vi "Main_02b.vi"() -> ()   [LabVIEW 2020]
uses:
  ENUM RPS Select.ctl
panel:
  in  "Example":string="A Y\nC Y\nC X\nA Y\nC X\nC Y\nB Z\nA Y\nA Y\nC Z\nA Y\nA Y\nA Y\nC Y\nA Y\nA Y\nA Y\nA X\nB X\nA X\nA Y\nC Y\nC X\nA Y\nA Y\nC Y\nA X\nA Y\nB Z\nA Y\nC X\nA Y\nA Y\nC Z\nC Y\nC X\nA Y\nA Z\nA Y\nA Y\nA Y\nA Y\nC Y\nC Y\nB Z\nB Z\nC Y\nB X\nA Y\nA Y\nA Y\nC Z\nA Y\nC X\nA Z\nC Y\nA Y\nA Y\nA Y\nA Y\nA Y\nC X\nA Y\nC Y\nA Y\nC Y\nA Y\nA X\nC Y\nA X\nA Y\nC Y\nC Y\nA Y\nC X\nA Y\nA Y\nA Y\nC X\nA Y\nA Y\nA Y\nC X\nA Y\nC X\nA Y\nA Y\nC Z\nA Y\nA Y\nA Y\nC X\nA Y\nA X\nC Y\nA X\nB Z\nC Y\nA Y\nA Y\nB Z\nC Y\nA Y\nA Z\nC Z\nC Y\nB Z\nA Y\nA Y\nC Y\nA Y\nC X\nA Y\nA Y\nC X\nC X\nC Y\nA Y\nA Y\nC X\nA Y\nA Y\nA Y\nA Y\nC X\nC Y\nA Y\nA Y\nA Y\nC Z\nA Y\nC Y\nA Y\nC X\nC Z\nA Y\nB X\nA Y\nC X\nA Y\nB X\nA Y\nC Z\nA Y\nA Y\nA Y\nA X\nA Y\nA Y\nA Y\nC Y\nA Y\nA Y\nA Y\nA Y\nC Y\nC X\nA Y\nA Y\nA Y\nA Y\nC Y\nA Y\nA Y\nA Y\nC Y\nB X\nA Y\nA Y\nA Y\nA Y\nA Y\nA X\nC Y\nA Y\nC X\nA X\nB Y\nA Y\nC X\nA Y\nC Y\nC Y\nA Z\nC Z\nC X\nB X\nC Y\nA Y\nC Z\nA Z\nA Y\nC X\nA Y\nA Y\nC X\nA Y\nB X\nC X\nA Z\nC Y\nA Y\nC X\nA Y\nA Y\nA Y\nB Z\nC Z\nA Y\nA X\nC X\nA Y\nA Y\nC Y\nA Y\nA Y\nA X\nA X\nC Y\nC X\nB X\nA Y\nA Y\nA Y\nA Y\nB Y\nA Y\nC Y\nA Y\nA X\nB Z\nA X\nC Z\nC X\nC X\nC Y\nC X\nC X\nA X\nC X\nA Y\nC Y\nA X\nC X\nB Z\nC Z\nA Y\nC X\nB Y\nA Z\nC Y\nC X\nA Y\nA Y\nA Y\nC X\nA Y\nA Y\nA Y\nA X\nB Y\nC Y\nC X\nB Z\nA Y\nA Y\nB Y\nA Y\nA Y\nA Y\nC X\nA Y\nA Y\nA Y\nA Y\nA Y\nA Y\nA Y\nA Y\nA Y\nC Y\nC Y\nC Z\nA Y\nC Y\nA Y\nA Y\nA X\nA X\nA Y\nA Y\nC Y\nA Y\nA X\nA Y\nA Y\nC X\nA Y\nC X\nC X\nC Y\nB Y\nA Y\nC X\nA Y\nA Y\nA X\nA Y\nA Y\nA X\nA Y\nB Z\nC Y\nA Y\nA Y\nA Y\nC Y\nC Z\nA Y\nA Y\nA Y\nA Y\nA Y\nC Y\nC Y\nC Y\nC Y\nC Y\nA X\nC Y\nA Y\nA Y\nA Y\nA Y\nC X\nA Y\nC Z\nA Y\nB Y\nA X\nA Y\nA Y\nA Y\nC Y\nC Y\nA X\nC Y\nA Y\nA Y\nA Y\nB Z\nA X\nA Y\nA Y\nA Z\nC Y\nA Y\nC X\nC Y\nC Y\nC Z\nB Y\nC X\nC X\nA Z\nC Y\nA Y\nA Z\nA X\nA Z\nC Y\nC X\nB Z\nA X\nC Y\nA Y\nC Y\nB Z\nA Y\nA Y\nC X\nC X\nC X\nA Y\nB X\nC X\nC Y\nC X\nA X\nA X\nB X\nA Y\nA Y\nA Y\nC X\nA Y\nC Y\nC X\nA Y\nB Z\nA Y\nA Y\nA Y\nB X\nA Y\nA Y\nA Y\nC Y\nA Y\nC X\nC Y\nC Y\nA Y\nB Z\nC Y\nC X\nC Y\nC X\nC X\nC Y\nA Y\nA Z\nA Y\nA Y\nA Y\nA Y\nC Z\nA Y\nA Y\nC Y\nA Y\nA X\nC Z\nC Y\nC X\nC X\nA Y\nA Z\nA Z\nB Y\nA X\nC X\nC X\nA Y\nA Y\nA Y\nC Z\nC X\nC X\nC X\nA Y\nC Z\nA Z\nC X\nC Y\nA X\nC X\nC X\nA Y\nC Y\nC Y\nB X\nB Z\nA Y\nA Y\nA Y\nB Z\nC Y\nA Y\nB Z\nA X\nC Y\nC Y\nB X\nC X\nB Y\nA Y\nB X\nC Z\nA Y\nA Z\nC Z\nC Z\nA Y\nA X\nA Y\nA X\nC Y\nA Y\nA Y\nA Y\nC X\nC X\nC X\nA Y\nA Y\nA Y\nA Y\nA Y\nC Y\nA Y\nC Y\nA Z\nC X\nC Y\nA Y\nA Y\nB Y\nC Y\nA Y\nC Z\nC Z\nA Y\nB Y\nA Y\nA Y\nA X\nC Y\nA Y\nA Y\nA Y\nC Z\nC Y\nC X\nA Y\nA Y\nB Z\nC Y\nC X\nC Z\nA Y\nC Y\nA Y\nA Y\nC X\nC Y\nC Y\nA Y\nC Y\nC X\nC Y\nA Y\nA Y\nA Y\nA Z\nB Z\nA Y\nA Y\nA X\nC Z\nC X\nA Y\nA Y\nA Y\nC X\nC Y\nB Z\nC X\nA Y\nA Y\nA Y\nC Y\nA Y\nC X\nC Z\nC X\nA Y\nA X\nA Y\nC Z\nC X\nB Y\nA Y\nA X\nA Y\nB Y\nA Y\nA Y\nC Y\nC Z\nC Y\nC Y\nC X\nA Y\nA Y\nA X\nA Y\nA Y\nA Z\nA X\nC Y\nA Y\nC Y\nC Y\nC Z\nC Y\nC Y\nA Z\nA Y\nC Z\nC Y\nC Y\nC Y\nB X\nC Y\nA Y\nC X\nA Y\nB X\nC Z\nC Z\nC Y\nA Y\nC X\nA Y\nA Y\nA Y\nA Y\nC Z\nA Z\nA X\nC Y\nC X\nA Y\nA Y\nC X\nC Y\nC Z\nC X\nC Y\nA X\nA Y\nA Y\nB X\nA Y\nA X\nC X\nA Y\nA Y\nA Y\nB Z\nA Z\nB Z\nC X\nB Z\nA Y\nC X\nA Y\nC X\nA Y\nA Y\nC Y\nA Y\nA Y\nB X\nA Y\nC Y\nA Y\nA Y\nA Y\nC Y\nA Y\nA Y\nA Y\nB Y\nA Y\nC Y\nA Y\nA Y\nA Y\nA Y\nC Y\nA X\nB X\nA Y\nB Z\nC X\nA X\nB X\nC Y\nA Y\nB X\nC Y\nA Y\nB X\nA Y\nC X\nB X\nA Y\nA Y\nA Y\nA Y\nC X\nC X\nA Y\nB X\nC Y\nA Y\nA Y\nA Y\nA Y\nB X\nA Y\nB Z\nC X\nA Y\nB Z\nC X\nC Z\nC Z\nB X\nC Y\nA Y\nA Y\nA Y\nA Y\nA Y\nA Y\nC Y\nA Y\nA Y\nA X\nA X\nC X\nA Y\nC Z\nC Y\nA Y\nC X\nA Z\nA Z\nA Y\nC Z\nA Y\nA Y\nA Y\nC Y\nA X\nC X\nC Z\nA Y\nA Y\nC X\nB X\nA Y\nA Z\nC Y\nA Z\nA Y\nA Y\nA Y\nA Y\nA Y\nB X\nA Y\nC Y\nC X\nA Y\nA Y\nC Z\nC Z\nC Y\nA Y\nB Z\nA Y\nA Y\nA Y\nA Y\nA Y\nC X\nA Z\nA Y\nC Y\nA Z\nC X\nA Y\nC X\nA Y\nA Y\nC Z\nC Y\nA Y\nA Z\nC X\nC X\nA Y\nB Z\nA Y\nB X\nC Y\nC X\nC Z\nA Y\nA X\nC X\nC Z\nC Y\nC X\nA Y\nA Y\nA Y\nA Y\nA Y\nA Y\nC Y\nA Y\nC Y\nA Y\nC Y\nB Y\nA Y\nA Y\nA Y\nA Y\nB Z\nC Y\nA Y\nC Y\nA X\nC Y\nA Y\nB Y\nC Y\nC X\nC X\nA Y\nA Y\nA Y\nC X\nA X\nA Y\nA X\nC Y\nA Y\nA Y\nC Y\nC Y\nA Z\nA Y\nA Y\nB X\nA Z\nB X\nA Y\nC Y\nA X\nC Y\nC Z\nB Z\nA Y\nA Y\nC Y\nA Y\nC Z\nA Y\nA X\nA Y\nC Y\nA Y\nA Y\nA Y\nA Y\nA Y\nA Y\nA Y\nA Y\nC X\nC Y\nA Y\nA Z\nA Y\nC X\nA Y\nC Z\nA Y\nC X\nA X\nA Y\nC Y\nA Y\nC X\nA X\nA Y\nA Y\nA Y\nC Y\nA Y\nC Y\nA Y\nB Y\nC Y\nC Y\nA Y\nA Y\nA Y\nA Y\nC Z\nA Y\nC Z\nA Y\nC Y\nB X\nA X\nC Y\nC Z\nA X\nA Z\nA Y\nA X\nC Z\nC Y\nA Z\nC Y\nA X\nA Y\nA Y\nA X\nC Z\nA X\nA Z\nC Y\nA Y\nC Y\nA Z\nB Z\nA Y\nC X\nC X\nA Y\nA Y\nA X\nA Y\nA Y\nA Y\nC X\nA Y\nB X\nA Y\nC X\nA Y\nC Y\nA Y\nC Y\nC Z\nC Y\nC Z\nA Z\nA Y\nC Y\nC Z\nC Z\nA Y\nA Y\nC Y\nA X\nA Y\nC Y\nA Y\nA Y\nA Y\nA X\nA Y\nB Z\nC Y\nC X\nA Y\nC X\nB X\nC Y\nC Y\nA Y\nC Y\nC Y\nA X\nA Y\nA X\nA Y\nA Z\nC Z\nB X\nA Y\nC X\nA Y\nC Z\nA Y\nC Y\nA Z\nA Y\nA Y\nA Y\nC Y\nC Y\nA Y\nA Y\nC Y\nA Y\nC Y\nC Y\nA X\nA Y\nC X\nC Z\nA Y\nA Y\nA Y\nC X\nC X\nC Y\nC Y\nC Z\nA X\nA Y\nC Y\nC Z\nA Y\nB Y\nA Y\nC Z\nC Z\nA Y\nA Y\nA Y\nB Z\nA Y\nA Z\nA X\nC X\nC X\nC Z\nA Y\nC Z\nA Z\nC Y\nC Z\nC X\nC Y\nC X\nA Y\nC Y\nA Z\nA Y\nA Y\nA Y\nA Y\nC Y\nA X\nC X\nA Y\nA Y\nC Z\nB Z\nA Y\nA Y\nC X\nA Y\nC Y\nC Y\nB Z\nA Y\nC Y\nA Y\nC X\nC X\nA Y\nC Y\nA X\nC X\nA Y\nC Z\nA Y\nC X\nA Y\nC X\nA Y\nC Y\nA Y\nC Z\nA Y\nC Z\nA Y\nA Y\nA Y\nC Y\nA Y\nA X\nA Z\nA Y\nC Y\nC Y\nA Y\nA Y\nB Z\nA X\nA X\nC X\nC X\nC Z\nC Z\nA Y\nA Y\nA Y\nA X\nA X\nA Y\nA Z\nC Y\nC Y\nC X\nA Y\nC X\nB X\nA X\nA Z\nA Y\nB X\nA Y\nB Z\nB Z\nA Y\nB X\nC Y\nA Y\nA Y\nC Y\nC Y\nA Y\nA Y\nA Z\nA Y\nC Z\nB X\nA Y\nC Y\nC Y\nA Y\nB X\nC X\nC Y\nA X\nC X\nA Y\nA X\nA Y\nA Y\nB Z\nA X\nC Y\nA Y\nA Z\nB Y\nA Y\nB X\nA Z\nC Y\nC Z\nC Z\nC Z\nC Y\nA Y\nC Y\nC Y\nB Y\nA Y\nC Z\nB Y\nA Y\nA Y\nA Y\nA X\nB Z\nA Y\nC Z\nA Y\nA X\nC Z\nC X\nA Y\nA Y\nA Y\nB Z\nB Z\nA Y\nC Z\nA Y\nA Y\nA Y\nC Y\nC Z\nC X\nA Y\nB Z\nC Y\nB Z\nC X\nC X\nA Y\nA X\nA X\nB Z\nC Y\nC Y\nC X\nA Y\nC X\nC X\nA Y\nC X\nC Z\nA X\nC Y\nC Y\nC Y\nA Y\nA X\nC Y\nA Y\nA Y\nC Y\nC X\nC Y\nB X\nC X\nA Z\nA X\nA Y\nC Y\nA Y\nA X\nC Y\nA Y\nA X\nC X\nA X\nC X\nC Y\nC Y\nA Y\nC X\nA Y\nA X\nC Y\nA Y\nC Z\nA Z\nA Y\nA Y\nA Y\nA Z\nA Y\nB X\nB Z\nC X\nA Z\nC X\nA Y\nA Z\nA X\nC Y\nC Y\nB Z\nA Z\nA Y\nA Y\nA Y\nB X\nC Y\nA Y\nA X\nA Y\nB Z\nB Z\nA Y\nA Y\nA Y\nC X\nC X\nC X\nC Y\nA Y\nC Y\nC Y\nA Y\nA Y\nA Y\nA Y\nC Y\nA Y\nC X\nA Y\nC X\nC Y\nC Y\nC Z\nB X\nA Y\nC Y\nA Y\nC Y\nA Y\nA Y\nA Y\nA Y\nB Z\nC Z\nC Y\nA X\nC Y\nA Y\nC Y\nC Y\nA Y\nB Z\nC Y\nB X\nB X\nA Y\nA Y\nC Y\nC Y\nB X\nA X\nC Y\nC X\nC Y\nA Y\nA Y\nC X\nA X\nA Z\nA Y\nA Z\nA Y\nB X\nA X\nC X\nA X\nC X\nC Z\nA Y\nC X\nC Y\nC X\nC Y\nA Y\nC Y\nA Y\nA Y\nC Y\nC Z\nC X\nA Y\nA Y\nA X\nC Y\nB Z\nA Y\nC Y\nB Z\nC Y\nA Y\nC Y\nA X\nA X\nA Y\nB X\nA Y\nC X\nC Y\nA Y\nA Y\nA Y\nC X\nC Z\nA Y\nC Y\nA Z\nC Y\nA Y\nC Y\nA Y\nC Z\nC Y\nC X\nA Y\nC X\nA Z\nB Z\nA Y\nA X\nA Y\nA Y\nA X\nA Y\nA Y\nA Y\nA Y\nC Y\nC X\nA Y\nA Y\nA Y\nA Y\nA Y\nC Y\nC Y\nC Y\nA X\nA Z\nA Y\nC X\nA Y\nA Y\nC Y\nB Y\nC Y\nA X\nA Y\nA Y\nA Y\nC X\nA X\nC Y\nC Z\nA Y\nB Z\nA Z\nC Y\nA Y\nA Y\nB Z\nA X\nA Y\nC Y\nA Y\nA X\nB X\nC Z\nB X\nA Y\nA Y\nC Y\nA Y\nA Z\nA Y\nA Y\nA Y\nC X\nA Y\nA Z\nA Z\nA Y\nC X\nA Y\nC Z\nC Y\nB X\nC Y\nA Y\nC Z\nB Z\nA Y\nC Y\nA Z\nA Y\nC X\nC Y\nA X\nA Y\nC Z\nA Y\nA Y\nA Y\nA Y\nB Z\nA Z\nC Z\nA X\nA Y\nA Y\nA Y\nA Y\nA Y\nC Y\nC Y\nA Y\nC X\nA Y\nA Y\nA X\nA X\nA Y\nC Y\nC Z\nA Z\nA Y\nA X\nB X\nB X\nB Z\nC X\nC Y\nA Y\nA Y\nA Y\nC Z\nA Y\nA Y\nA Y\nC Y\nC Y\nB Y\nC Z\nB Z\nC Y\nB Z\nA Y\nA X\nC X\nA X\nC X\nB Y\nA Y\nA Z\nA Y\nA X\nA Y\nA Y\nC X\nA Y\nA Y\nC X\nC X\nA Y\nC X\nC Z\nC X\nB Z\nB Z\nB Z\nC Y\nB Z\nC Y\nC Z\nB Y\nA Y\nC Z\nA Y\nC X\nC X\nB Z\nB Y\nA Y\nA Z\nC Y\nC X\nC Y\nA Z\nC X\nC X\nC X\nA Y\nA Y\nC Y\nA Y\nC Y\nC Y\nA Y\nC Y\nC Z\nA Y\nB Y\nC Y\nC X\nA Y\nA Y\nA X\nA Y\nC Y\nB Z\nA Y\nA Y\nA Y\nA Y\nC X\nB X\nA Y\nA Y\nA Y\nA Y\nB X\nA Y\nA Y\nA X\nC Y\nA Y\nA Y\nC X\nA Y\nA Y\nA Y\nC X\nB Y\nA Z\nC Y\nC X\nA Y\nA Z\nB X\nA Y\nA Y\nA X\nC Y\nC Y\nC Y\nA Y\nC Z\nA Y\nA Y\nC Y\nB Z\nA Y\nA Y\nC X\nA X\nA Y\nA Y\nA Y\nB Z\nC Y\nA Y\nC Y\nC Y\nA Y\nA Y\nC Y\nC Y\nA Y\nC Y\nA Y\nB X\nC Y\nA X\nA Z\nA Y\nA Y\nC Y\nC Y\nA Y\nC Z\nA Z\nA Y\nA Y\nC Y\nC Y\nC X\nC Y\nA Y\nC X\nC Y\nA Y\nC X\nC Y\nC Y\nA Y\nA Y\nA Y\nC X\nC Y\nA Y\nA Y\nC Y\nA Y\nC Y\nA Y\nA Y\nC Y\nC Y\nC Y\nA Z\nA Y\nC Y\nC Y\nA Y\nA X\nC X\nA Y\nC Y\nB X\nC Y\nA Y\nA Y\nC Y\nC Y\nA Y\nA Y\nA Y\nB Z\nA Y\nC Y\nA Y\nA Y\nC X\nC Y\nA Y\nA Y\nC Y\nC Y\nC Y\nC Z\nA Y\nA Y\nC X\nA Y\nC Z\nA X\nC X\nB X\nA Y\nC Y\nA Y\nA Y\nA X\nA Y\nA Z\nB Y\nA X\nA Y\nC Y\nC Y\nC X\nA Y\nC Y\nA Y\nC Y\nA Y\nC X\nC X\nA Y\nC Y\nC Z\nC X\nB X\nA Y\nB X\nA Y\nA Y\nC Y\nA Y\nC Y\nA Y\nA Y\nA Y\nA Y\nA X\nA Z\nA Y\nB X\nA Y\nA Y\nC X\nA Y\nC Z\nA Y\nA Y\nC Y\nC X\nC X\nA Y\nA Y\nB X\nC X\nA Y\nC Y\nA Y\nC Y\nA Y\nB Z\nA Y\nC Y\nA Y\nA Y\nA Y\nC Z\nA Y\nA X\nC X\nA X\nA Y\nA Y\nA Y\nC X\nC Y\nC Y\nC Y\nA Y\nA Y\nA Z\nC X\nA Y\nA Y\nA Y\nC Y\nC Y\nA X\nA Y\nC Y\nB Y\nA Y\nA Z\nC X\nA Y\nA Z\nA X\nA Y\nA Y\nA Y\nC Y\nA Y\nA Y\nA X\nC Y\nA X\nB X\nC X\nC Y\nA Y\nA Y\nA Y\nC Y\nA Y\nA Y\nA Y\nA X\nC X\nA Y\nA Y\nA Y\nC Y\nA Y\nB Y\nC Y\nC Y\nC Y\nC Y\nA Y\nA Y\nC Y\nC Y\nA Y\nC Y\nC Y\nA Y\nC Y\nC X\nC X\nC Y\nA X\nC X\nC X\nA Z\nC Y\nC Z\nA Y\nB Z\nA Y\nA Y\nB X\nC Y\nA Y\nC Z\nA Y\nC Z\nA Y\nA Y\nA X\nC Y\nC X\nC X\nC Y\nC X\nA Y\nA Y\nC X\nA Y\nA Z\nB X\nC X\nC Y\nB X\nB Z\nA Y\nA Y\nA Y\nC Y\nA X\nC Y\nC Y\nC X\nA Y\nC X\nA Y\nA X\nC X\nA Y\nA Y\nA X\nC Y\nB Y\nA Y\nA X\nA Y\nC Y\nA X\nC Y\nA Z\nA Y\nA Y\nC Z\nA Z\nC Y\nA Y\nC Y\nA Y\nA Z\nC Y\nC Y\nB Z\nB Y\nC X\nC X\nB Z\nA Y\nA Y\nA Y\nA Y\nA Y\nA Y\nC X\nA Y\nC Y\nA Y\nB Y\nA Y\nA Y\nB X\nA X\nC X\nC Y\nA Y\nC Y\nA Y\nA Y\nA Y\nA Y\nC X\nB Z\nA Z\nC Y\nB Y\nC X\nA Y\nA X\nA Y\nA Y\nC Y\nC Y\nA Y\nA Y\nC Y\nB Z\nC Y\nA X\nC Y\nA Z\nA Y\nA Y\nA Y\nB X\nA Y\nC Y\nC X\nB Y\nC Y\nA Y\nB Y\nA Y\nA Y\nC X\nC Y\nC Y\nA Y\nA Y\nC X\nC X\nC Y\nA Y\nC X\nC X\nB X\nC Y\nA Y\nC Y\nB Z\nA Y\nB X\nC Y\nC X\nA X\nA Y\nC Y\nA Y\nA Y\nA Y\nC X\nA Y\nC X\nC X\nA Y\nC Y\nA Y\nB Z\nC X\nC Y\nC Y\nB X\nA Y\nC Y\nA X\nA X\nB Z\nC X\nA Y\nC Y\nA Y\nA X\nC Y\nA Y\nA Y\nA X\nA X\nA Z\nC Z\nB Y\nC Y\nC X\nA Y\nA Y\nC Y\nA Y\nC Z\nC X\nC X\nC Z\nC Y\nC X\nC X\nA Y\nC Z\nB X\nC Z\nA Y\nA Y\nC Y\nC X\nC Z\nC X\nC X\nC Y\nC X\nC Y\nA Y\nA X\nA Y\nC X\nA Y\nA Y\nA Y\nA Y\nA Z\nC X\nA X\nB X\nA Y\nA Y\nC Z\nC Y\nA Y\nA Y\nC Y\nC Y\nC Y\nA Y\nA Y\nA Y\nB X\nA Y\nB Z\nA Z\nA X\nA X\nC Y\nA Y\nC Z\nA Y\nA Y\nC Y\nA Y\nA X\nC Y\nC Y\nA X\nA Y\nC Y\nA Y\nC X\nA Y\nC X\nA X\nA Y\nA Y\nA Y\nB X\nC Z\nA Z\nB Y\nA Y\nB Z\nB Z\nA Y\nC Z\nB Z\nA Y\nA Y\nA Y\nC Y\nB X\nA Y\nC X\nA Y\nC Z\nC X\nB Y\nC X\nC X\nB X\nC Y\nB Z\nA X\nA Y\nB Y\nC Z\nA Y\nA Z\nA Y\nC X\nA Y\nA Y\nC Y\nC X\nB Y\nB X\nC Y\nB X\nC Y\nA X\nA Z\nA X\nC X\nB Z\nC Y\nC X\nA Y\nA Y\nA X\nB X\nC X\nA Y\nB Y\nC Z\nA Y\nC Y\nA Y\nA Y\nA Y\nB X\nA Y\nC X\nA Y\nA Y\nA Y\nA X\nC X\nA X\nC Z\nC Y\nA Y\nA Y\nC Y\nA X\nC Z\nA Y\nA Y\nA Y\nB Y\nC Y\nC Y\nC Z\nC Z\nC Z\nA Y\nC Y\nA Y\nA Y\nA Y\nA Y\nA Y\nB Y\nC Y\nC Y\nA X\nC Z\nC Y\nA Y\nA Y\nA Y\nC X\nA Z\nA Y\nA Y\nA X\nA Z\nC X\nB Y\nA Y\nA Y\nC Y\nB X\nA Y\nA Y\nC Y\nC Y\nC Z\nA X\nC Y\nC X\nC X\nC Z\nA X\nB Z\nC X\nC X\nC Y\nC X\nC Z\nC X\nC X\nB Z\nB Z\nA Y\nB Z\nA Y\nA Y\nA Y\nB X\nC X\nA Y\nC Z\nA Z\nA X\nA Y\nB Y\nB X\nB Z\nA Y\nA X\nA X\nA Y\nC X\nB X\nA Y\nC Y\nA Y\nA Y\nC X\nC Y\nC X\nC Z\nB X\nC X\nC Z\nA Z\nA X\nA Y\nA Y\nA Y\nC Z\nA Y\nC Y\nC X\nA Y\nA Y\nC X\nC X\nA Y\nC Y\nC Z\nC Y\nC X\nB Y\nC Y\nC X\nA Y\nB X\nC X\nA Y\nA Y\nC Y\nC Z\nA Y\nA Z\nB Y\nA Y\nB X\nC Y\nC Z\nB X\nB X\nC X\nA Y\nB Z\nA Y\nA Y\nA Y\nA Y\nC X\nA Y\nA Y\nC Z\nC X\nB Y\nC Y\nC Y\nA Y\nC X\nB Z\nA Z\nC Y\nA Y\nB Y\nB X\nB Y\nA Z\nC Y\nC Z\nA Y\nC Z\nC X\nA Y\nA Z\nC Z\nA Y\nA Y\nA Y\nC X\nA Y\nC Y\nB Z\nA Y\nC X\nA X\nA Y\nC Y\nC Z\nC Y\nA Y\nC Z\nA Z\nA Y\nC Y\nA Y\nC X\nA Y\nA Y\nB Z\nA Y\nA Y\nA Y\nC Y\nC Y\nC Y\nC X\nC Y\nC X\nB Z\nA Y\nA Y\nA Z\nA Z\nA Y\nA Z\nA Y\nA Y\nA X\nC Z\nA Y\nA Y\nA Y\nC X\nC Y\nC X\nA Y\nA Y\nA Y\nC Y\nC X\nB Y\nA Y\nC Y\nC Y\nA Z\nC Z\nA Y\nA X\nA Y\nA Y\nB X\nA Y\nC Y\nA X\nC Y\nA Y\nA Y\nA X\nC Y\nA X\nB X\nC Y\nA Y\nA Y\nA Y\nA Y\nC Z\nC Y\nC X\nA X\nA Y\nC X\nC Y\nA X\nA X\nB Y\nB Z\nA Y\nC Z\nA X\nC Y\nA X\nA Y\nC Y\nC X\nC Y\nC X\nA Y\nA X\nA Y\nA X\nC Z\nA X\nA Y\nC Y\nC X\nC Y\nC X\nA Y\nC Y\nC X\nA Y\nA Y\nC Y\nC Y\nA Y\nA Z\nC Y\nA Z\nA Y\nC Y\nA Y\nA Y\nC Y\nA Y\nB X\nC X\nC Y\nC X\nA Y\nB Y\nC Z\nA Y\nC X\nA Y"
  out "Score":u32
  in  "Puzzle":string="A Y\nC Y\nC X\nA Y\nC X\nC Y\nB Z\nA Y\nA Y\nC Z\nA Y\nA Y\nA Y\nC Y\nA Y\nA Y\nA Y\nA X\nB X\nA X\nA Y\nC Y\nC X\nA Y\nA Y\nC Y\nA X\nA Y\nB Z\nA Y\nC X\nA Y\nA Y\nC Z\nC Y\nC X\nA Y\nA Z\nA Y\nA Y\nA Y\nA Y\nC Y\nC Y\nB Z\nB Z\nC Y\nB X\nA Y\nA Y\nA Y\nC Z\nA Y\nC X\nA Z\nC Y\nA Y\nA Y\nA Y\nA Y\nA Y\nC X\nA Y\nC Y\nA Y\nC Y\nA Y\nA X\nC Y\nA X\nA Y\nC Y\nC Y\nA Y\nC X\nA Y\nA Y\nA Y\nC X\nA Y\nA Y\nA Y\nC X\nA Y\nC X\nA Y\nA Y\nC Z\nA Y\nA Y\nA Y\nC X\nA Y\nA X\nC Y\nA X\nB Z\nC Y\nA Y\nA Y\nB Z\nC Y\nA Y\nA Z\nC Z\nC Y\nB Z\nA Y\nA Y\nC Y\nA Y\nC X\nA Y\nA Y\nC X\nC X\nC Y\nA Y\nA Y\nC X\nA Y\nA Y\nA Y\nA Y\nC X\nC Y\nA Y\nA Y\nA Y\nC Z\nA Y\nC Y\nA Y\nC X\nC Z\nA Y\nB X\nA Y\nC X\nA Y\nB X\nA Y\nC Z\nA Y\nA Y\nA Y\nA X\nA Y\nA Y\nA Y\nC Y\nA Y\nA Y\nA Y\nA Y\nC Y\nC X\nA Y\nA Y\nA Y\nA Y\nC Y\nA Y\nA Y\nA Y\nC Y\nB X\nA Y\nA Y\nA Y\nA Y\nA Y\nA X\nC Y\nA Y\nC X\nA X\nB Y\nA Y\nC X\nA Y\nC Y\nC Y\nA Z\nC Z\nC X\nB X\nC Y\nA Y\nC Z\nA Z\nA Y\nC X\nA Y\nA Y\nC X\nA Y\nB X\nC X\nA Z\nC Y\nA Y\nC X\nA Y\nA Y\nA Y\nB Z\nC Z\nA Y\nA X\nC X\nA Y\nA Y\nC Y\nA Y\nA Y\nA X\nA X\nC Y\nC X\nB X\nA Y\nA Y\nA Y\nA Y\nB Y\nA Y\nC Y\nA Y\nA X\nB Z\nA X\nC Z\nC X\nC X\nC Y\nC X\nC X\nA X\nC X\nA Y\nC Y\nA X\nC X\nB Z\nC Z\nA Y\nC X\nB Y\nA Z\nC Y\nC X\nA Y\nA Y\nA Y\nC X\nA Y\nA Y\nA Y\nA X\nB Y\nC Y\nC X\nB Z\nA Y\nA Y\nB Y\nA Y\nA Y\nA Y\nC X\nA Y\nA Y\nA Y\nA Y\nA Y\nA Y\nA Y\nA Y\nA Y\nC Y\nC Y\nC Z\nA Y\nC Y\nA Y\nA Y\nA X\nA X\nA Y\nA Y\nC Y\nA Y\nA X\nA Y\nA Y\nC X\nA Y\nC X\nC X\nC Y\nB Y\nA Y\nC X\nA Y\nA Y\nA X\nA Y\nA Y\nA X\nA Y\nB Z\nC Y\nA Y\nA Y\nA Y\nC Y\nC Z\nA Y\nA Y\nA Y\nA Y\nA Y\nC Y\nC Y\nC Y\nC Y\nC Y\nA X\nC Y\nA Y\nA Y\nA Y\nA Y\nC X\nA Y\nC Z\nA Y\nB Y\nA X\nA Y\nA Y\nA Y\nC Y\nC Y\nA X\nC Y\nA Y\nA Y\nA Y\nB Z\nA X\nA Y\nA Y\nA Z\nC Y\nA Y\nC X\nC Y\nC Y\nC Z\nB Y\nC X\nC X\nA Z\nC Y\nA Y\nA Z\nA X\nA Z\nC Y\nC X\nB Z\nA X\nC Y\nA Y\nC Y\nB Z\nA Y\nA Y\nC X\nC X\nC X\nA Y\nB X\nC X\nC Y\nC X\nA X\nA X\nB X\nA Y\nA Y\nA Y\nC X\nA Y\nC Y\nC X\nA Y\nB Z\nA Y\nA Y\nA Y\nB X\nA Y\nA Y\nA Y\nC Y\nA Y\nC X\nC Y\nC Y\nA Y\nB Z\nC Y\nC X\nC Y\nC X\nC X\nC Y\nA Y\nA Z\nA Y\nA Y\nA Y\nA Y\nC Z\nA Y\nA Y\nC Y\nA Y\nA X\nC Z\nC Y\nC X\nC X\nA Y\nA Z\nA Z\nB Y\nA X\nC X\nC X\nA Y\nA Y\nA Y\nC Z\nC X\nC X\nC X\nA Y\nC Z\nA Z\nC X\nC Y\nA X\nC X\nC X\nA Y\nC Y\nC Y\nB X\nB Z\nA Y\nA Y\nA Y\nB Z\nC Y\nA Y\nB Z\nA X\nC Y\nC Y\nB X\nC X\nB Y\nA Y\nB X\nC Z\nA Y\nA Z\nC Z\nC Z\nA Y\nA X\nA Y\nA X\nC Y\nA Y\nA Y\nA Y\nC X\nC X\nC X\nA Y\nA Y\nA Y\nA Y\nA Y\nC Y\nA Y\nC Y\nA Z\nC X\nC Y\nA Y\nA Y\nB Y\nC Y\nA Y\nC Z\nC Z\nA Y\nB Y\nA Y\nA Y\nA X\nC Y\nA Y\nA Y\nA Y\nC Z\nC Y\nC X\nA Y\nA Y\nB Z\nC Y\nC X\nC Z\nA Y\nC Y\nA Y\nA Y\nC X\nC Y\nC Y\nA Y\nC Y\nC X\nC Y\nA Y\nA Y\nA Y\nA Z\nB Z\nA Y\nA Y\nA X\nC Z\nC X\nA Y\nA Y\nA Y\nC X\nC Y\nB Z\nC X\nA Y\nA Y\nA Y\nC Y\nA Y\nC X\nC Z\nC X\nA Y\nA X\nA Y\nC Z\nC X\nB Y\nA Y\nA X\nA Y\nB Y\nA Y\nA Y\nC Y\nC Z\nC Y\nC Y\nC X\nA Y\nA Y\nA X\nA Y\nA Y\nA Z\nA X\nC Y\nA Y\nC Y\nC Y\nC Z\nC Y\nC Y\nA Z\nA Y\nC Z\nC Y\nC Y\nC Y\nB X\nC Y\nA Y\nC X\nA Y\nB X\nC Z\nC Z\nC Y\nA Y\nC X\nA Y\nA Y\nA Y\nA Y\nC Z\nA Z\nA X\nC Y\nC X\nA Y\nA Y\nC X\nC Y\nC Z\nC X\nC Y\nA X\nA Y\nA Y\nB X\nA Y\nA X\nC X\nA Y\nA Y\nA Y\nB Z\nA Z\nB Z\nC X\nB Z\nA Y\nC X\nA Y\nC X\nA Y\nA Y\nC Y\nA Y\nA Y\nB X\nA Y\nC Y\nA Y\nA Y\nA Y\nC Y\nA Y\nA Y\nA Y\nB Y\nA Y\nC Y\nA Y\nA Y\nA Y\nA Y\nC Y\nA X\nB X\nA Y\nB Z\nC X\nA X\nB X\nC Y\nA Y\nB X\nC Y\nA Y\nB X\nA Y\nC X\nB X\nA Y\nA Y\nA Y\nA Y\nC X\nC X\nA Y\nB X\nC Y\nA Y\nA Y\nA Y\nA Y\nB X\nA Y\nB Z\nC X\nA Y\nB Z\nC X\nC Z\nC Z\nB X\nC Y\nA Y\nA Y\nA Y\nA Y\nA Y\nA Y\nC Y\nA Y\nA Y\nA X\nA X\nC X\nA Y\nC Z\nC Y\nA Y\nC X\nA Z\nA Z\nA Y\nC Z\nA Y\nA Y\nA Y\nC Y\nA X\nC X\nC Z\nA Y\nA Y\nC X\nB X\nA Y\nA Z\nC Y\nA Z\nA Y\nA Y\nA Y\nA Y\nA Y\nB X\nA Y\nC Y\nC X\nA Y\nA Y\nC Z\nC Z\nC Y\nA Y\nB Z\nA Y\nA Y\nA Y\nA Y\nA Y\nC X\nA Z\nA Y\nC Y\nA Z\nC X\nA Y\nC X\nA Y\nA Y\nC Z\nC Y\nA Y\nA Z\nC X\nC X\nA Y\nB Z\nA Y\nB X\nC Y\nC X\nC Z\nA Y\nA X\nC X\nC Z\nC Y\nC X\nA Y\nA Y\nA Y\nA Y\nA Y\nA Y\nC Y\nA Y\nC Y\nA Y\nC Y\nB Y\nA Y\nA Y\nA Y\nA Y\nB Z\nC Y\nA Y\nC Y\nA X\nC Y\nA Y\nB Y\nC Y\nC X\nC X\nA Y\nA Y\nA Y\nC X\nA X\nA Y\nA X\nC Y\nA Y\nA Y\nC Y\nC Y\nA Z\nA Y\nA Y\nB X\nA Z\nB X\nA Y\nC Y\nA X\nC Y\nC Z\nB Z\nA Y\nA Y\nC Y\nA Y\nC Z\nA Y\nA X\nA Y\nC Y\nA Y\nA Y\nA Y\nA Y\nA Y\nA Y\nA Y\nA Y\nC X\nC Y\nA Y\nA Z\nA Y\nC X\nA Y\nC Z\nA Y\nC X\nA X\nA Y\nC Y\nA Y\nC X\nA X\nA Y\nA Y\nA Y\nC Y\nA Y\nC Y\nA Y\nB Y\nC Y\nC Y\nA Y\nA Y\nA Y\nA Y\nC Z\nA Y\nC Z\nA Y\nC Y\nB X\nA X\nC Y\nC Z\nA X\nA Z\nA Y\nA X\nC Z\nC Y\nA Z\nC Y\nA X\nA Y\nA Y\nA X\nC Z\nA X\nA Z\nC Y\nA Y\nC Y\nA Z\nB Z\nA Y\nC X\nC X\nA Y\nA Y\nA X\nA Y\nA Y\nA Y\nC X\nA Y\nB X\nA Y\nC X\nA Y\nC Y\nA Y\nC Y\nC Z\nC Y\nC Z\nA Z\nA Y\nC Y\nC Z\nC Z\nA Y\nA Y\nC Y\nA X\nA Y\nC Y\nA Y\nA Y\nA Y\nA X\nA Y\nB Z\nC Y\nC X\nA Y\nC X\nB X\nC Y\nC Y\nA Y\nC Y\nC Y\nA X\nA Y\nA X\nA Y\nA Z\nC Z\nB X\nA Y\nC X\nA Y\nC Z\nA Y\nC Y\nA Z\nA Y\nA Y\nA Y\nC Y\nC Y\nA Y\nA Y\nC Y\nA Y\nC Y\nC Y\nA X\nA Y\nC X\nC Z\nA Y\nA Y\nA Y\nC X\nC X\nC Y\nC Y\nC Z\nA X\nA Y\nC Y\nC Z\nA Y\nB Y\nA Y\nC Z\nC Z\nA Y\nA Y\nA Y\nB Z\nA Y\nA Z\nA X\nC X\nC X\nC Z\nA Y\nC Z\nA Z\nC Y\nC Z\nC X\nC Y\nC X\nA Y\nC Y\nA Z\nA Y\nA Y\nA Y\nA Y\nC Y\nA X\nC X\nA Y\nA Y\nC Z\nB Z\nA Y\nA Y\nC X\nA Y\nC Y\nC Y\nB Z\nA Y\nC Y\nA Y\nC X\nC X\nA Y\nC Y\nA X\nC X\nA Y\nC Z\nA Y\nC X\nA Y\nC X\nA Y\nC Y\nA Y\nC Z\nA Y\nC Z\nA Y\nA Y\nA Y\nC Y\nA Y\nA X\nA Z\nA Y\nC Y\nC Y\nA Y\nA Y\nB Z\nA X\nA X\nC X\nC X\nC Z\nC Z\nA Y\nA Y\nA Y\nA X\nA X\nA Y\nA Z\nC Y\nC Y\nC X\nA Y\nC X\nB X\nA X\nA Z\nA Y\nB X\nA Y\nB Z\nB Z\nA Y\nB X\nC Y\nA Y\nA Y\nC Y\nC Y\nA Y\nA Y\nA Z\nA Y\nC Z\nB X\nA Y\nC Y\nC Y\nA Y\nB X\nC X\nC Y\nA X\nC X\nA Y\nA X\nA Y\nA Y\nB Z\nA X\nC Y\nA Y\nA Z\nB Y\nA Y\nB X\nA Z\nC Y\nC Z\nC Z\nC Z\nC Y\nA Y\nC Y\nC Y\nB Y\nA Y\nC Z\nB Y\nA Y\nA Y\nA Y\nA X\nB Z\nA Y\nC Z\nA Y\nA X\nC Z\nC X\nA Y\nA Y\nA Y\nB Z\nB Z\nA Y\nC Z\nA Y\nA Y\nA Y\nC Y\nC Z\nC X\nA Y\nB Z\nC Y\nB Z\nC X\nC X\nA Y\nA X\nA X\nB Z\nC Y\nC Y\nC X\nA Y\nC X\nC X\nA Y\nC X\nC Z\nA X\nC Y\nC Y\nC Y\nA Y\nA X\nC Y\nA Y\nA Y\nC Y\nC X\nC Y\nB X\nC X\nA Z\nA X\nA Y\nC Y\nA Y\nA X\nC Y\nA Y\nA X\nC X\nA X\nC X\nC Y\nC Y\nA Y\nC X\nA Y\nA X\nC Y\nA Y\nC Z\nA Z\nA Y\nA Y\nA Y\nA Z\nA Y\nB X\nB Z\nC X\nA Z\nC X\nA Y\nA Z\nA X\nC Y\nC Y\nB Z\nA Z\nA Y\nA Y\nA Y\nB X\nC Y\nA Y\nA X\nA Y\nB Z\nB Z\nA Y\nA Y\nA Y\nC X\nC X\nC X\nC Y\nA Y\nC Y\nC Y\nA Y\nA Y\nA Y\nA Y\nC Y\nA Y\nC X\nA Y\nC X\nC Y\nC Y\nC Z\nB X\nA Y\nC Y\nA Y\nC Y\nA Y\nA Y\nA Y\nA Y\nB Z\nC Z\nC Y\nA X\nC Y\nA Y\nC Y\nC Y\nA Y\nB Z\nC Y\nB X\nB X\nA Y\nA Y\nC Y\nC Y\nB X\nA X\nC Y\nC X\nC Y\nA Y\nA Y\nC X\nA X\nA Z\nA Y\nA Z\nA Y\nB X\nA X\nC X\nA X\nC X\nC Z\nA Y\nC X\nC Y\nC X\nC Y\nA Y\nC Y\nA Y\nA Y\nC Y\nC Z\nC X\nA Y\nA Y\nA X\nC Y\nB Z\nA Y\nC Y\nB Z\nC Y\nA Y\nC Y\nA X\nA X\nA Y\nB X\nA Y\nC X\nC Y\nA Y\nA Y\nA Y\nC X\nC Z\nA Y\nC Y\nA Z\nC Y\nA Y\nC Y\nA Y\nC Z\nC Y\nC X\nA Y\nC X\nA Z\nB Z\nA Y\nA X\nA Y\nA Y\nA X\nA Y\nA Y\nA Y\nA Y\nC Y\nC X\nA Y\nA Y\nA Y\nA Y\nA Y\nC Y\nC Y\nC Y\nA X\nA Z\nA Y\nC X\nA Y\nA Y\nC Y\nB Y\nC Y\nA X\nA Y\nA Y\nA Y\nC X\nA X\nC Y\nC Z\nA Y\nB Z\nA Z\nC Y\nA Y\nA Y\nB Z\nA X\nA Y\nC Y\nA Y\nA X\nB X\nC Z\nB X\nA Y\nA Y\nC Y\nA Y\nA Z\nA Y\nA Y\nA Y\nC X\nA Y\nA Z\nA Z\nA Y\nC X\nA Y\nC Z\nC Y\nB X\nC Y\nA Y\nC Z\nB Z\nA Y\nC Y\nA Z\nA Y\nC X\nC Y\nA X\nA Y\nC Z\nA Y\nA Y\nA Y\nA Y\nB Z\nA Z\nC Z\nA X\nA Y\nA Y\nA Y\nA Y\nA Y\nC Y\nC Y\nA Y\nC X\nA Y\nA Y\nA X\nA X\nA Y\nC Y\nC Z\nA Z\nA Y\nA X\nB X\nB X\nB Z\nC X\nC Y\nA Y\nA Y\nA Y\nC Z\nA Y\nA Y\nA Y\nC Y\nC Y\nB Y\nC Z\nB Z\nC Y\nB Z\nA Y\nA X\nC X\nA X\nC X\nB Y\nA Y\nA Z\nA Y\nA X\nA Y\nA Y\nC X\nA Y\nA Y\nC X\nC X\nA Y\nC X\nC Z\nC X\nB Z\nB Z\nB Z\nC Y\nB Z\nC Y\nC Z\nB Y\nA Y\nC Z\nA Y\nC X\nC X\nB Z\nB Y\nA Y\nA Z\nC Y\nC X\nC Y\nA Z\nC X\nC X\nC X\nA Y\nA Y\nC Y\nA Y\nC Y\nC Y\nA Y\nC Y\nC Z\nA Y\nB Y\nC Y\nC X\nA Y\nA Y\nA X\nA Y\nC Y\nB Z\nA Y\nA Y\nA Y\nA Y\nC X\nB X\nA Y\nA Y\nA Y\nA Y\nB X\nA Y\nA Y\nA X\nC Y\nA Y\nA Y\nC X\nA Y\nA Y\nA Y\nC X\nB Y\nA Z\nC Y\nC X\nA Y\nA Z\nB X\nA Y\nA Y\nA X\nC Y\nC Y\nC Y\nA Y\nC Z\nA Y\nA Y\nC Y\nB Z\nA Y\nA Y\nC X\nA X\nA Y\nA Y\nA Y\nB Z\nC Y\nA Y\nC Y\nC Y\nA Y\nA Y\nC Y\nC Y\nA Y\nC Y\nA Y\nB X\nC Y\nA X\nA Z\nA Y\nA Y\nC Y\nC Y\nA Y\nC Z\nA Z\nA Y\nA Y\nC Y\nC Y\nC X\nC Y\nA Y\nC X\nC Y\nA Y\nC X\nC Y\nC Y\nA Y\nA Y\nA Y\nC X\nC Y\nA Y\nA Y\nC Y\nA Y\nC Y\nA Y\nA Y\nC Y\nC Y\nC Y\nA Z\nA Y\nC Y\nC Y\nA Y\nA X\nC X\nA Y\nC Y\nB X\nC Y\nA Y\nA Y\nC Y\nC Y\nA Y\nA Y\nA Y\nB Z\nA Y\nC Y\nA Y\nA Y\nC X\nC Y\nA Y\nA Y\nC Y\nC Y\nC Y\nC Z\nA Y\nA Y\nC X\nA Y\nC Z\nA X\nC X\nB X\nA Y\nC Y\nA Y\nA Y\nA X\nA Y\nA Z\nB Y\nA X\nA Y\nC Y\nC Y\nC X\nA Y\nC Y\nA Y\nC Y\nA Y\nC X\nC X\nA Y\nC Y\nC Z\nC X\nB X\nA Y\nB X\nA Y\nA Y\nC Y\nA Y\nC Y\nA Y\nA Y\nA Y\nA Y\nA X\nA Z\nA Y\nB X\nA Y\nA Y\nC X\nA Y\nC Z\nA Y\nA Y\nC Y\nC X\nC X\nA Y\nA Y\nB X\nC X\nA Y\nC Y\nA Y\nC Y\nA Y\nB Z\nA Y\nC Y\nA Y\nA Y\nA Y\nC Z\nA Y\nA X\nC X\nA X\nA Y\nA Y\nA Y\nC X\nC Y\nC Y\nC Y\nA Y\nA Y\nA Z\nC X\nA Y\nA Y\nA Y\nC Y\nC Y\nA X\nA Y\nC Y\nB Y\nA Y\nA Z\nC X\nA Y\nA Z\nA X\nA Y\nA Y\nA Y\nC Y\nA Y\nA Y\nA X\nC Y\nA X\nB X\nC X\nC Y\nA Y\nA Y\nA Y\nC Y\nA Y\nA Y\nA Y\nA X\nC X\nA Y\nA Y\nA Y\nC Y\nA Y\nB Y\nC Y\nC Y\nC Y\nC Y\nA Y\nA Y\nC Y\nC Y\nA Y\nC Y\nC Y\nA Y\nC Y\nC X\nC X\nC Y\nA X\nC X\nC X\nA Z\nC Y\nC Z\nA Y\nB Z\nA Y\nA Y\nB X\nC Y\nA Y\nC Z\nA Y\nC Z\nA Y\nA Y\nA X\nC Y\nC X\nC X\nC Y\nC X\nA Y\nA Y\nC X\nA Y\nA Z\nB X\nC X\nC Y\nB X\nB Z\nA Y\nA Y\nA Y\nC Y\nA X\nC Y\nC Y\nC X\nA Y\nC X\nA Y\nA X\nC X\nA Y\nA Y\nA X\nC Y\nB Y\nA Y\nA X\nA Y\nC Y\nA X\nC Y\nA Z\nA Y\nA Y\nC Z\nA Z\nC Y\nA Y\nC Y\nA Y\nA Z\nC Y\nC Y\nB Z\nB Y\nC X\nC X\nB Z\nA Y\nA Y\nA Y\nA Y\nA Y\nA Y\nC X\nA Y\nC Y\nA Y\nB Y\nA Y\nA Y\nB X\nA X\nC X\nC Y\nA Y\nC Y\nA Y\nA Y\nA Y\nA Y\nC X\nB Z\nA Z\nC Y\nB Y\nC X\nA Y\nA X\nA Y\nA Y\nC Y\nC Y\nA Y\nA Y\nC Y\nB Z\nC Y\nA X\nC Y\nA Z\nA Y\nA Y\nA Y\nB X\nA Y\nC Y\nC X\nB Y\nC Y\nA Y\nB Y\nA Y\nA Y\nC X\nC Y\nC Y\nA Y\nA Y\nC X\nC X\nC Y\nA Y\nC X\nC X\nB X\nC Y\nA Y\nC Y\nB Z\nA Y\nB X\nC Y\nC X\nA X\nA Y\nC Y\nA Y\nA Y\nA Y\nC X\nA Y\nC X\nC X\nA Y\nC Y\nA Y\nB Z\nC X\nC Y\nC Y\nB X\nA Y\nC Y\nA X\nA X\nB Z\nC X\nA Y\nC Y\nA Y\nA X\nC Y\nA Y\nA Y\nA X\nA X\nA Z\nC Z\nB Y\nC Y\nC X\nA Y\nA Y\nC Y\nA Y\nC Z\nC X\nC X\nC Z\nC Y\nC X\nC X\nA Y\nC Z\nB X\nC Z\nA Y\nA Y\nC Y\nC X\nC Z\nC X\nC X\nC Y\nC X\nC Y\nA Y\nA X\nA Y\nC X\nA Y\nA Y\nA Y\nA Y\nA Z\nC X\nA X\nB X\nA Y\nA Y\nC Z\nC Y\nA Y\nA Y\nC Y\nC Y\nC Y\nA Y\nA Y\nA Y\nB X\nA Y\nB Z\nA Z\nA X\nA X\nC Y\nA Y\nC Z\nA Y\nA Y\nC Y\nA Y\nA X\nC Y\nC Y\nA X\nA Y\nC Y\nA Y\nC X\nA Y\nC X\nA X\nA Y\nA Y\nA Y\nB X\nC Z\nA Z\nB Y\nA Y\nB Z\nB Z\nA Y\nC Z\nB Z\nA Y\nA Y\nA Y\nC Y\nB X\nA Y\nC X\nA Y\nC Z\nC X\nB Y\nC X\nC X\nB X\nC Y\nB Z\nA X\nA Y\nB Y\nC Z\nA Y\nA Z\nA Y\nC X\nA Y\nA Y\nC Y\nC X\nB Y\nB X\nC Y\nB X\nC Y\nA X\nA Z\nA X\nC X\nB Z\nC Y\nC X\nA Y\nA Y\nA X\nB X\nC X\nA Y\nB Y\nC Z\nA Y\nC Y\nA Y\nA Y\nA Y\nB X\nA Y\nC X\nA Y\nA Y\nA Y\nA X\nC X\nA X\nC Z\nC Y\nA Y\nA Y\nC Y\nA X\nC Z\nA Y\nA Y\nA Y\nB Y\nC Y\nC Y\nC Z\nC Z\nC Z\nA Y\nC Y\nA Y\nA Y\nA Y\nA Y\nA Y\nB Y\nC Y\nC Y\nA X\nC Z\nC Y\nA Y\nA Y\nA Y\nC X\nA Z\nA Y\nA Y\nA X\nA Z\nC X\nB Y\nA Y\nA Y\nC Y\nB X\nA Y\nA Y\nC Y\nC Y\nC Z\nA X\nC Y\nC X\nC X\nC Z\nA X\nB Z\nC X\nC X\nC Y\nC X\nC Z\nC X\nC X\nB Z\nB Z\nA Y\nB Z\nA Y\nA Y\nA Y\nB X\nC X\nA Y\nC Z\nA Z\nA X\nA Y\nB Y\nB X\nB Z\nA Y\nA X\nA X\nA Y\nC X\nB X\nA Y\nC Y\nA Y\nA Y\nC X\nC Y\nC X\nC Z\nB X\nC X\nC Z\nA Z\nA X\nA Y\nA Y\nA Y\nC Z\nA Y\nC Y\nC X\nA Y\nA Y\nC X\nC X\nA Y\nC Y\nC Z\nC Y\nC X\nB Y\nC Y\nC X\nA Y\nB X\nC X\nA Y\nA Y\nC Y\nC Z\nA Y\nA Z\nB Y\nA Y\nB X\nC Y\nC Z\nB X\nB X\nC X\nA Y\nB Z\nA Y\nA Y\nA Y\nA Y\nC X\nA Y\nA Y\nC Z\nC X\nB Y\nC Y\nC Y\nA Y\nC X\nB Z\nA Z\nC Y\nA Y\nB Y\nB X\nB Y\nA Z\nC Y\nC Z\nA Y\nC Z\nC X\nA Y\nA Z\nC Z\nA Y\nA Y\nA Y\nC X\nA Y\nC Y\nB Z\nA Y\nC X\nA X\nA Y\nC Y\nC Z\nC Y\nA Y\nC Z\nA Z\nA Y\nC Y\nA Y\nC X\nA Y\nA Y\nB Z\nA Y\nA Y\nA Y\nC Y\nC Y\nC Y\nC X\nC Y\nC X\nB Z\nA Y\nA Y\nA Z\nA Z\nA Y\nA Z\nA Y\nA Y\nA X\nC Z\nA Y\nA Y\nA Y\nC X\nC Y\nC X\nA Y\nA Y\nA Y\nC Y\nC X\nB Y\nA Y\nC Y\nC Y\nA Z\nC Z\nA Y\nA X\nA Y\nA Y\nB X\nA Y\nC Y\nA X\nC Y\nA Y\nA Y\nA X\nC Y\nA X\nB X\nC Y\nA Y\nA Y\nA Y\nA Y\nC Z\nC Y\nC X\nA X\nA Y\nC X\nC Y\nA X\nA X\nB Y\nB Z\nA Y\nC Z\nA X\nC Y\nA X\nA Y\nC Y\nC X\nC Y\nC X\nA Y\nA X\nA Y\nA X\nC Z\nA X\nA Y\nC Y\nC X\nC Y\nC X\nA Y\nC Y\nC X\nA Y\nA Y\nC Y\nC Y\nA Y\nA Z\nC Y\nA Z\nA Y\nC Y\nA Y\nA Y\nC Y\nA Y\nB X\nC X\nC Y\nC X\nA Y\nB Y\nC Z\nA Y\nC X\nA Y"
  # "--- Part Two ---\nThe Elf finishes helping with the tent and sneaks back over to you. \"Anyway, the second column says how the round needs to end: X means you need to lose, Y means you need to end the round in a draw, and Z means you need to win. Good luck!\"\n\nThe total score is still calculated in the same way, but now you need to figure out what shape to choose so the round ends as indicated. The example above now goes like this:\n\nIn the first round, your opponent will choose Rock (A), and you need the round to end in a draw (Y), so you also choose Rock. This gives you a score of 1 + 3 = 4.\nIn the second round, your opponent will choose Paper (B), and you choose Rock so you lose (X) with a score of 1 + 0 = 1.\nIn the third round, you will defeat your opponent's Scissors with Rock for a score of 1 + 6 = 7.\nNow that you're correctly decrypting the ultra top secret strategy guide, you would get a total score of 12.\n\nFollowing the Elf's instructions for the second column, what would your total score be if everything goes exactly according to your strategy guide?"
  # "11258"
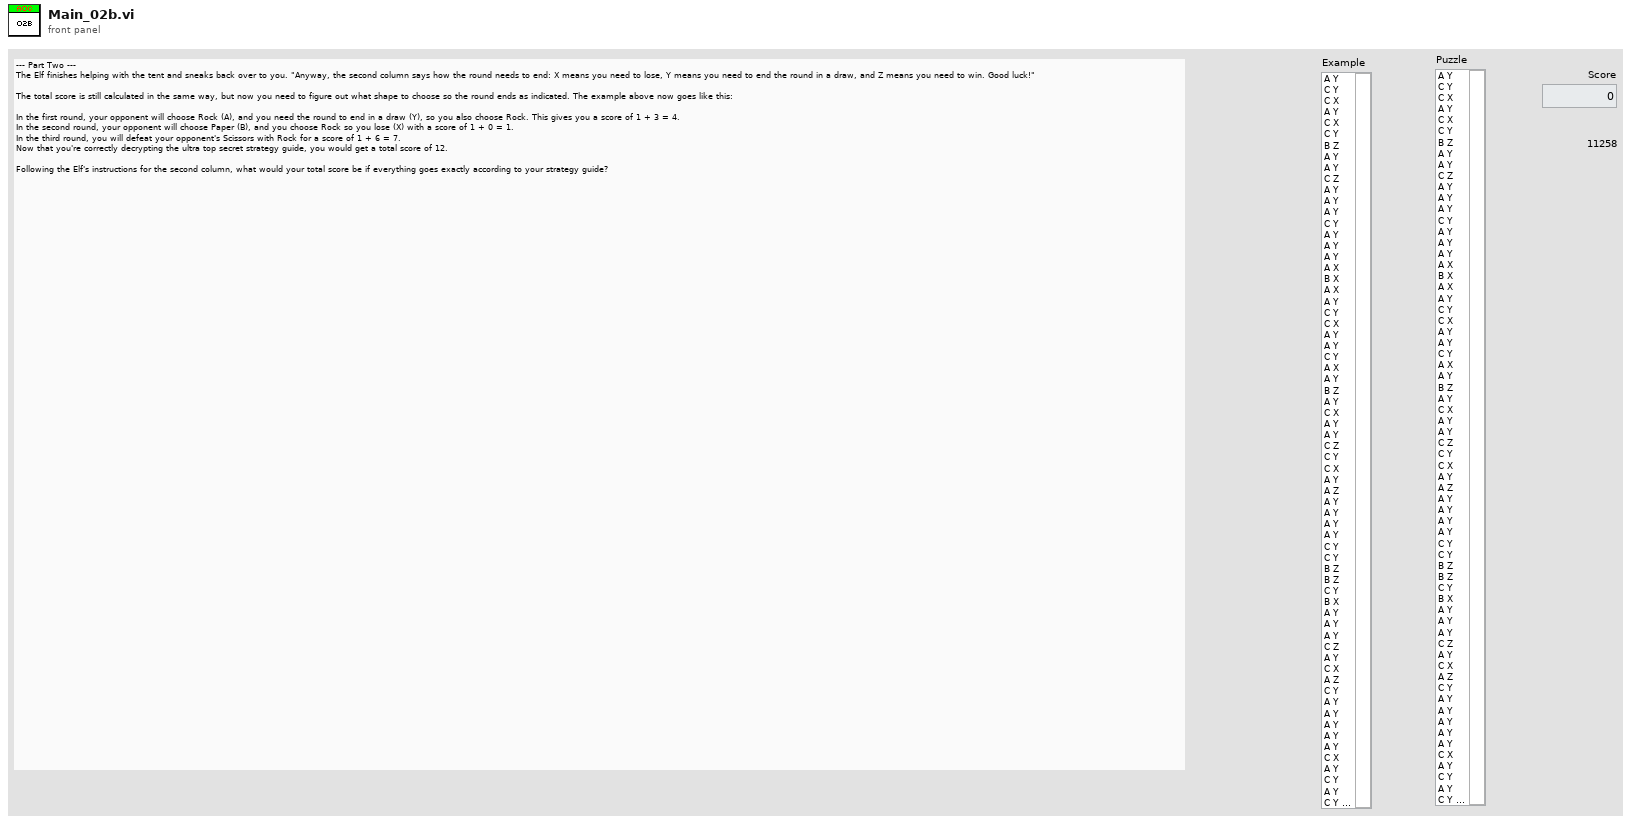
[diagram p1: front panel]
types:
  T1 = typedef "ENUM RPS Select.ctl" = enum16{"A", "B", "C", "X", "Y", "Z"}
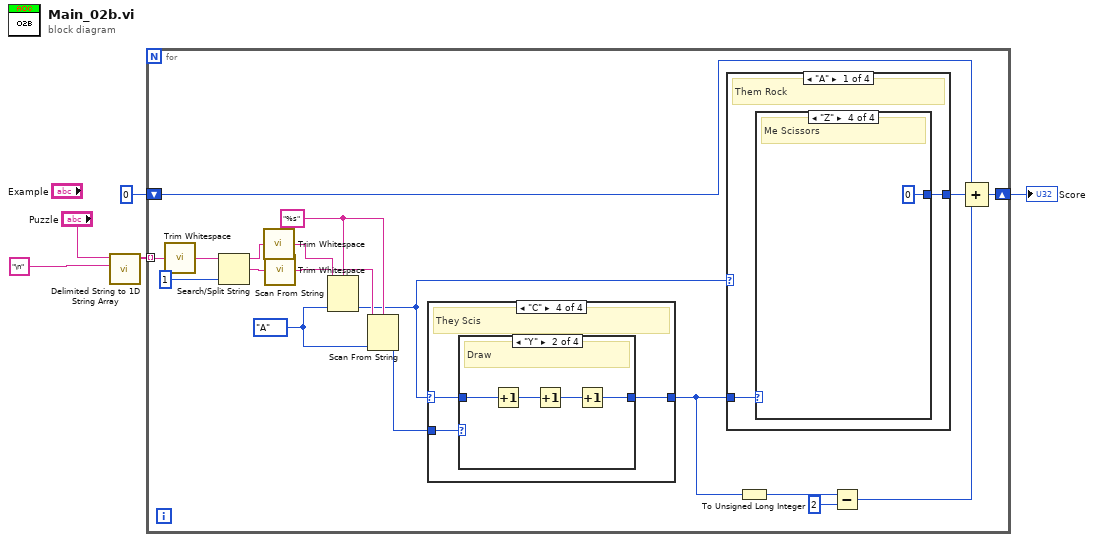
[diagram p0: block diagram]
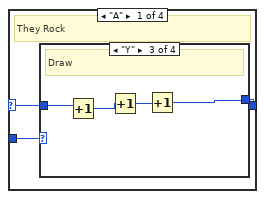
[diagram p2: hidden frame]
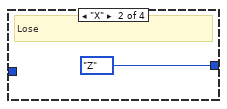
[diagram p4: hidden frame]
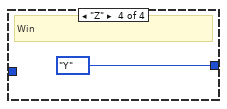
[diagram p5: hidden frame]
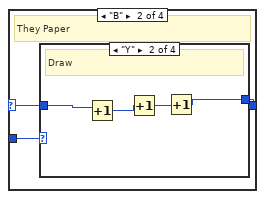
[diagram p6: hidden frame]
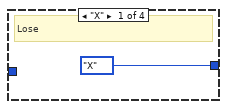
[diagram p7: hidden frame]
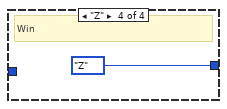
[diagram p9: hidden frame]
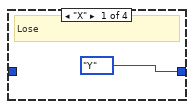
[diagram p11: hidden frame]
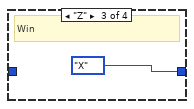
[diagram p12: hidden frame]
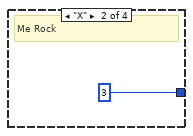
[diagram p15: hidden frame]
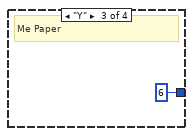
[diagram p16: hidden frame]
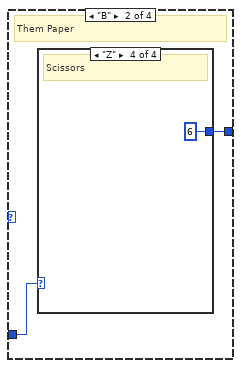
[diagram p17: hidden frame]
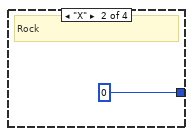
[diagram p19: hidden frame]
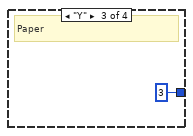
[diagram p20: hidden frame]
diagram:
  n1 = call <vilib>:"Delimited String to 1D String Array.vi"("delimiter"="\n", "delimited string"="Puzzle") -> ("string array"=w4:string[])  [unwired: 9 in]
  n2 = for {
    tunnel: w4 -> [w23] mode=indexing
    shift-right: [w14] -> w3
    shift-left: u32 0 -> [w13]
    w19 = "%s" ("format string")
    w20 = ENUM_RPS_Select."A" ("Select")
    n3 = call <vilib>:"Trim Whitespace.vi"("string"=w23) -> ("trimmed string"=w21:string)  [unwired: 1 in]
    n4 = Search/Split String(string=w21, offset (0)=1) -> (substring before match=w18:string, match + rest of string=w16:string)  [unwired: 1 in, 1 out]
    n5 = call <vilib>:"Trim Whitespace.vi"("string"=w18) -> ("trimmed string"=w17:string)  [unwired: 1 in]
    n6 = call <vilib>:"Trim Whitespace.vi"("string"=w16) -> ("trimmed string"=w15:string)  [unwired: 1 in]
    n7 = Scan From String(format string=w19, input string=w17, default 1=w20) -> (output 1=w8:T1)  [unwired: 2 in, 3 out]
    n8 = Scan From String(format string=w19, input string=w15, default 1=w20) -> (output 1=w10:T1)  [unwired: 2 in, 3 out]
    n9 = case shown="\"C\"" w8 {
      selector: w8 -> [w24 w33 _ w42]
      tunnel: w10 -> [w26 w35 _ w44]
      tunnel: [w25 w34 _ w43] -> w9
      frame "A" {
        # "They Rock"
        n10 = case shown="\"Y\"" w26 {
          tunnel: [_ ENUM_RPS_Select."Z" ("Select") w28 ENUM_RPS_Select."Y" ("Select")] -> w25
          tunnel: w24 -> [_ _ w31 _]
          frame Default {
          }
          frame "X" {
            # "Lose"
          }
          frame "Y" {
            # "Draw"
            n11 = Increment(x=w31) -> (x+1=w29:T1)
            n12 = Increment(x=w29) -> (x+1=w30:T1)
            n13 = Increment(x=w30) -> (x+1=w28:T1)
          }
          frame "Z" {
            # "Win"
          }
        }
      }
      frame "B" {
        # "They Paper"
        n14 = case shown="\"Y\"" w35 {
          tunnel: [ENUM_RPS_Select."X" ("Select") w37 _ ENUM_RPS_Select."Z" ("Select")] -> w34
          tunnel: w33 -> [_ w38 _ _]
          frame "X" {
            # "Lose"
          }
          frame "Y" {
            # "Draw"
            n15 = Increment(x=w38) -> (x+1=w39:T1)
            n16 = Increment(x=w39) -> (x+1=w40:T1)
            n17 = Increment(x=w40) -> (x+1=w37:T1)
          }
          frame Default {
          }
          frame "Z" {
            # "Win"
          }
        }
      }
      frame Default {
      }
      frame "C" {
        # "They Scis"
        n18 = case shown="\"Y\"" w44 {
          tunnel: [ENUM_RPS_Select."Y" ("Select") w46 ENUM_RPS_Select."X" ("Select") _] -> w43
          tunnel: w42 -> [_ w47 _ _]
          frame "X" {
            # "Lose"
          }
          frame "Y" {
            # "Draw"
            n19 = Increment(x=w47) -> (x+1=w48:T1)
            n20 = Increment(x=w48) -> (x+1=w49:T1)
            n21 = Increment(x=w49) -> (x+1=w46:T1)
          }
          frame "Z" {
            # "Win"
          }
          frame Default {
          }
        }
      }
    }
    n22 = case shown="\"A\"" w8 {
      tunnel: w9 -> [w52 w57 w62 _]
      tunnel: [w51 w56 w61 _] -> w6
      frame "A" {
        # "Them Rock"
        n23 = case shown="\"Z\"" w52 {
          tunnel: [_ u32 3 u32 6 u32 0] -> w51
          frame "A".."C" {
          }
          frame "X" {
            # "Me Rock"
          }
          frame "Y" {
            # "Me Paper"
          }
          frame "Z" {
            # "Me Scissors"
          }
        }
      }
      frame "B" {
        # "Them Paper"
        n24 = case shown="\"Z\"" w57 {
          tunnel: [_ u32 0 u32 3 u32 6] -> w56
          frame "A".."C" {
          }
          frame "X" {
            # "Rock"
          }
          frame "Y" {
            # "Paper"
          }
          frame "Z" {
            # "Scissors"
          }
        }
      }
      frame "C" {
        # "Them Scissors"
        n25 = case shown="\"Z\"" w62 {
          tunnel: [_ u32 6 u32 0 u32 3] -> w61
          frame "A".."C" {
          }
          frame "X" {
            # "Rock"
          }
          frame "Y" {
            # "Paper"
          }
          frame "Z" {
            # "Scissors"
          }
        }
      }
      frame "X".."Z" {
      }
    }
    n26 = To Unsigned Long Integer(number=w9) -> (unsigned 32bit integer=w12:u32)
    n27 = Subtract(x=w12, y=u32 2) -> (x-y=w7:u32)
    n28 = Compound Arithmetic op=ADD(w13, w6, w7) -> (w14:u32)
  }
  "Score" <- w3
